vi "2 WaypointHeadingGoodness.vi"(4 "Heading to Test":dbl) -> (1 "Goodness":dbl)   [LabVIEW 2011]
doc: "Takes the absolute wind vector, the heading of your next waypoint, and your current heading, and recommends a heading.\n\nWe repeatedly run the iterate theta VI until its outputs converge. The converging outputs are the two angles which minimize the travel time to the waypoint.\n\nAfter the while loop, we determine which angle is closer to the current heading. We choose the closer heading unless the other heading has a significantly higher dr/dt."
uses:
  2 Globals/2 Global.vi
  2 Classes/Waypoint/Waypoint.lvclass
panel:
  in  "Waypoint East":dbl
  in  "Waypoint North":dbl
  in  "Wind Angle":dbl
  # "Inputs"
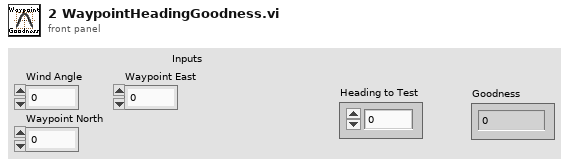
[diagram p1: front panel]
types:
  T1 = typedef "Velocity.ctl" = cluster{"East":dbl, "North":dbl}
  T2 = typedef "UTM Location.ctl" = cluster{"UTM Zone":dbl, "Hemisphere":enum16{"North", "South"}, "East":dbl, "North":dbl}
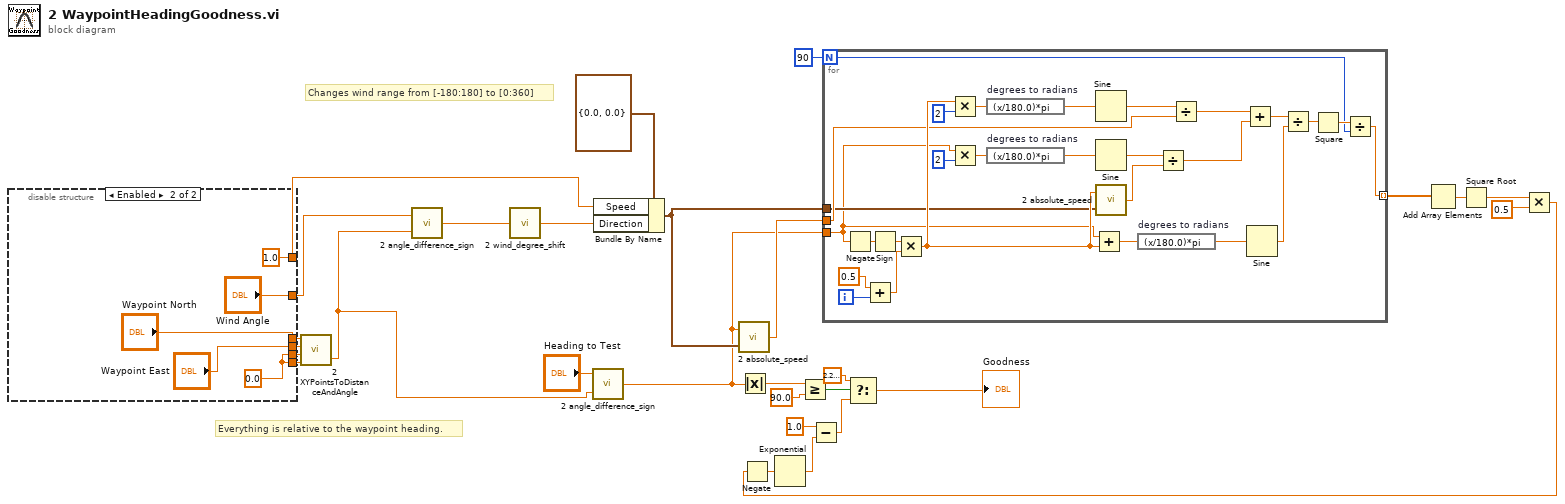
[diagram p0: block diagram]
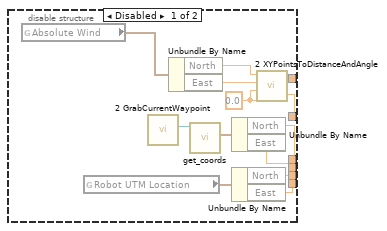
[diagram p2: hidden frame]
diagram:
  # "Changes wind range from [-180:180] to [0:360]"
  # "Everything is relative to the waypoint heading."
  n1 = disable-structure shown="Enabled" {
    disable-tunnel: [w35 "Wind Angle"] -> w10
    disable-tunnel: [w34 1.0 ("Distance")] -> w9
    disable-tunnel: [w33 w45] -> w8
    disable-tunnel: [w32 w45] -> w7
    disable-tunnel: [w31 "Waypoint North"] -> w6
    disable-tunnel: [w30 "Waypoint East"] -> w5
    frame Disabled {
      w36 = 0.0
      n2 = global read "2 Global.vi" "Absolute Wind"() -> (w39:T1)
      n3 = global read "2 Global.vi" "Robot UTM Location"() -> (w40:T2)
      n4 = call "2 GrabCurrentWaypoint.vi"() -> ("Current Waypoint"=w42:refnum<class "Waypoint.lvclass">)  [unwired: 11 in]
      n5 = Unbundle By Name(w39) -> ("North"=w37:dbl, "East"=w38:dbl)
      n6 = call-dynamic "get_coords.vi"("Waypoint in"=w42) -> ("Coords"=w41:T2)  [unwired: 7 in, 3 out]
      n7 = Unbundle By Name(w41) -> ("North"=w31:dbl, "East"=w30:dbl)
      n8 = Unbundle By Name(w40) -> ("North"=w32:dbl, "East"=w33:dbl)
      n9 = call "2 XYPointsToDistanceAndAngle.vi"("East 2"=w36, "North 2"=w36, "East 1"=w38, "North 1"=w37) -> ("Angle Diff"=w35:dbl, "Distance"=w34:dbl)
    }
    frame Enabled {
      w45 = 0.0 ("Distance")
    }
  }
  n10 = call "2 XYPointsToDistanceAndAngle.vi"("East 2"=w8, "North 2"=w7, "East 1"=w5, "North 1"=w6) -> ("Angle Diff"=w25:dbl)  [unwired: 1 out]
  n11 = call "2 angle_difference_sign.vi"("Angle 2"=w25, "Angle 1"=w10) -> ("Difference"=w29:dbl)
  n12 = call "2 wind_degree_shift.vi"("Wind Theta -180 - 180"=w29) -> ("Wind Theta 0-360"=w28:dbl)
  n13 = call "2 angle_difference_sign.vi"("Angle 2"=w25, "Angle 1"="Heading to Test") -> ("Difference"=w13:dbl)
  n14 = Bundle By Name(cluster=cluster{"Speed":dbl, "Direction":dbl} {"Speed"=0.0, "Direction"=0.0} ("input cluster"), "Speed"=w9, "Direction"=w28) -> (w14:cluster{"Speed":dbl, "Direction":dbl})
  n15 = call "2 absolute_speed.vi"("Wind Vector"=w14, "Boat Angle"=w13) -> ("Velocity"=w15:dbl)
  n16 = Absolute Value(x=w13) -> (abs(x)=w21:dbl)
  n17 = Greater Or Equal?(x=w21, y=90.0) -> (x >= y?=w23:bool)
  n18 = for {
    N: 90 -> [w53]
    tunnel: w15 -> [w63]
    tunnel: w14 -> [w49]
    tunnel: w13 -> [w48]
    tunnel: [w55] -> w4 mode=indexing
    i -> [w51]
    n19 = Negate(x=w48) -> (-x=w74:dbl)
    n20 = Add(x=0.5, y=w51) -> (x+y=w50:dbl)
    n21 = Sign(1:w74) -> (0:w75:dbl)
    n22 = Multiply(x=w75, y=w50) -> (x*y=w65:dbl)
    n23 = Multiply(x=w65, y=2) -> (x*y=w68:dbl)
    n24 = Multiply(x=w48, y=2) -> (x*y=w69:dbl)
    n25 = expression code="(x/180.0)*pi" "degrees to radians"(w68) -> (w66:dbl)
    n26 = expression code="(x/180.0)*pi" "degrees to radians"(w69) -> (w73:dbl)
    n27 = Add(x=w48, y=w65) -> (x+y=w70:dbl)
    n28 = Sine(x=w66) -> (sin(x)=w64:dbl)
    n29 = Sine(x=w73) -> (sin(x)=w62:dbl)
    n30 = call "2 absolute_speed.vi"("Wind Vector"=w49, "Boat Angle"=w65) -> ("Velocity"=w61:dbl)
    n31 = expression code="(x/180.0)*pi" "degrees to radians"(w70) -> (w71:dbl)
    n32 = Divide(x=w62, y=w61) -> (x/y=w59:dbl)
    n33 = Divide(x=w64, y=w63) -> (x/y=w60:dbl)
    n34 = Add(x=w60, y=w59) -> (x+y=w58:dbl)
    n35 = Sine(x=w71) -> (sin(x)=w57:dbl)
    n36 = Divide(x=w58, y=w57) -> (x/y=w56:dbl)
    n37 = Square(x=w56) -> (x^2=w54:dbl)
    n38 = Divide(x=w54, y=w53) -> (x/y=w55:dbl)
  }
  n39 = Add Array Elements(numeric array=w4) -> (sum=w11:dbl)
  n40 = Square Root(x=w11) -> (sqrt(x)=w1:dbl)
  n41 = Multiply(x=w1, y=0.5) -> (x*y=w2:dbl)
  n42 = Negate(x=w2) -> (-x=w17:dbl)
  n43 = Exponential(1:w17) -> (0:w18:dbl)
  n44 = Subtract(x=1.0, y=w18) -> (x-y=w16:dbl)
  n45 = Select(t=2.220446049250313e-16, s=w23, f=w16) -> (s? t:f=→"Goodness":dbl)
